vi "Litho objects manager.vi"() -> ()   [LabVIEW 2016]
uses:
  D:/Labview/Yang Hu/nanowriting_Akash/subVIs/Global Variables.vi
panel:
  in  "Cluster 2":T1
  in  "Cluster":T2
  in  "OK":bool
  in  "error in (no error)":errorcluster
  in  "Object index":string[](array[string])=["p6"]
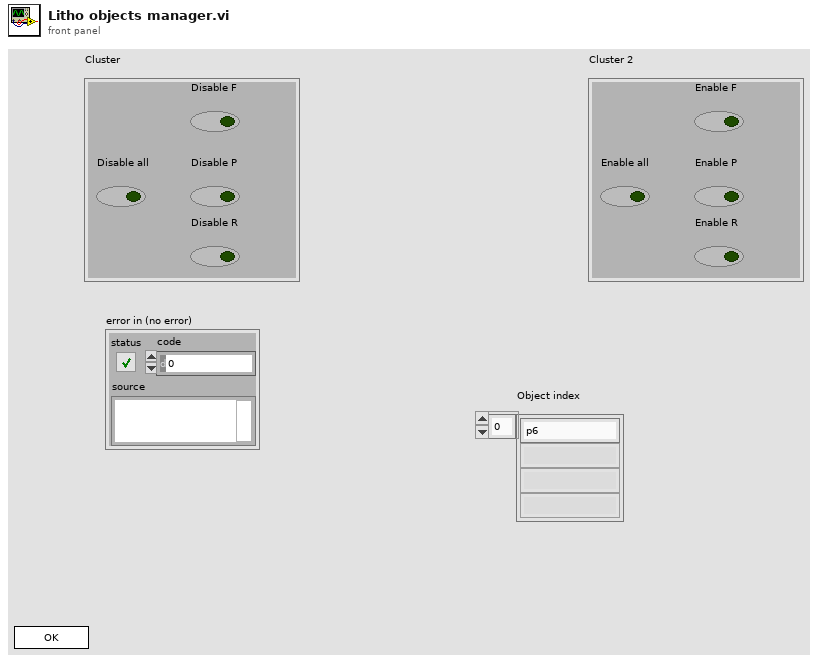
[diagram p1: front panel]
types:
  T1 = cluster{"Enable all":bool, "Enable F":bool, "Enable P":bool, "Enable R":bool}
  T2 = cluster{"Disable all":bool, "Disable F":bool, "Disable P":bool, "Disable R":bool}
  T3 = typedef "Funnel Properties - cluster.ctl" = cluster{"Enabled":bool, "Direction":u16, "Smooth Segments":dbl, "Bottom Segs.":dbl, "Speed (um/s)":T4, "Voltage (V)":T4, "Set Resistance":T7}
  T4 = typedef "Voltage - cluster.ctl" = cluster{"Schedule":T5, "Value":dbl, "Start Value":dbl, "End Value":dbl, "Min Value":dbl, "Max Value":dbl, "Duty Cycle (%)":dbl, "Signal Type":T6, "Cycle Number":dbl, "Phase (degrees)":dbl, "formula":string, "formula length (nm)":dbl, "formula resolution (nm)":dbl}
  T5 = typedef "Schedule - enum.ctl" = enum16{"Constant", "Ramp", "Fn. Generator", "Formula"}
  T6 = typedef "Signal Type - enum.ctl" = enum16{"Sine Wave", "Triangle Wave", "Square Wave", "Sawtooth Wave"}
  T7 = typedef "Resistor--enum.ctl" = enum16{"open", "discharge tip", "0 ohms", "100k ohm", "10M ohm", "1G ohm"}
  T8 = typedef "Path Properties - cluster.ctl" = cluster{"Enabled":bool, "Direction":u16, "Fill Orientation":u16, "Smooth Segments":dbl, "Fill Spacing":dbl, "Speed (um/s)":T4, "Voltage (V)":T4, "Set Resistance":T7}
  T9 = typedef "Rectangle Properties - cluster.ctl" = cluster{"Enabled":bool, "Direction":u16, "Fill Orientation":u16, "Fill Spacing":dbl, "Speed (um/s)":T4, "Voltage (V)":T4, "Set Resistance":T7}
  T10 = enum32{"Invalid", "Standard", "Closed", "Hidden", "Minimized", "Maximized"}
  T11 = enum32{"invalid app kind", "Development System", "Run Time System", "Student Edition", "Embedded LabVIEW", "Evaluation", "Custom"}
  T12 = cluster{"Core":cluster{"Current VI Reference":refnum<vi>, "Close Panel on Exit?":bool}, "Your Boolean data":bool, "Your string data":string}
  T13 = cluster{"Current VI Reference":refnum<vi>, "Close Panel on Exit?":bool}
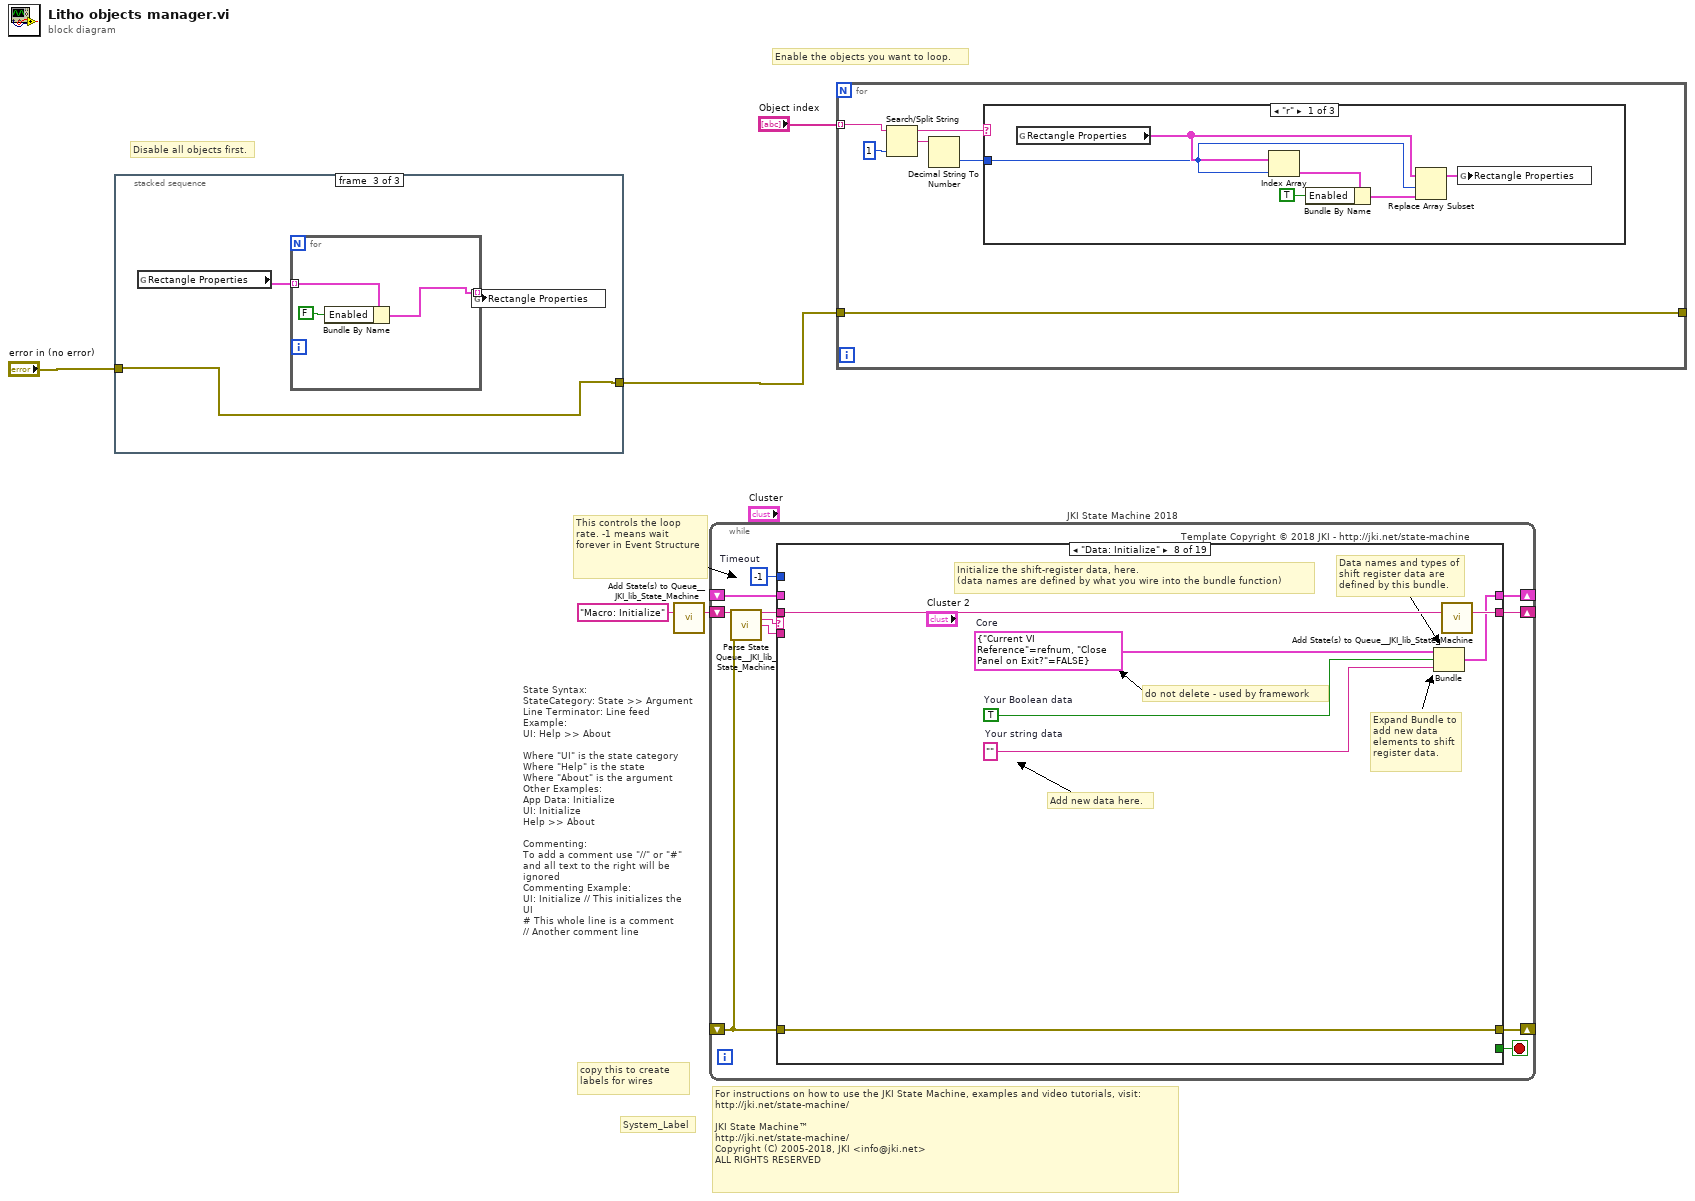
[diagram p0: block diagram]
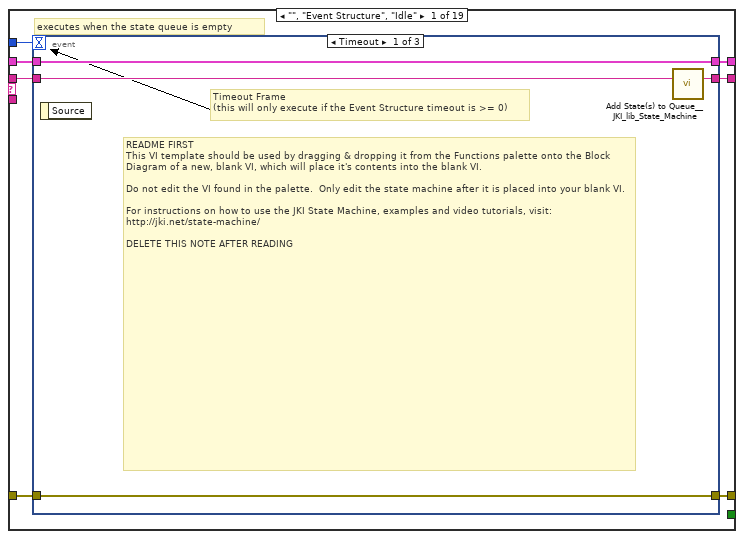
[diagram p2: hidden frame]
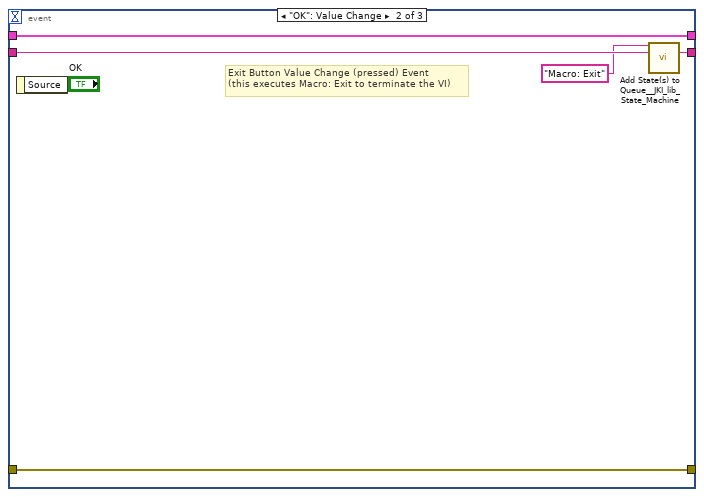
[diagram p3: hidden frame]
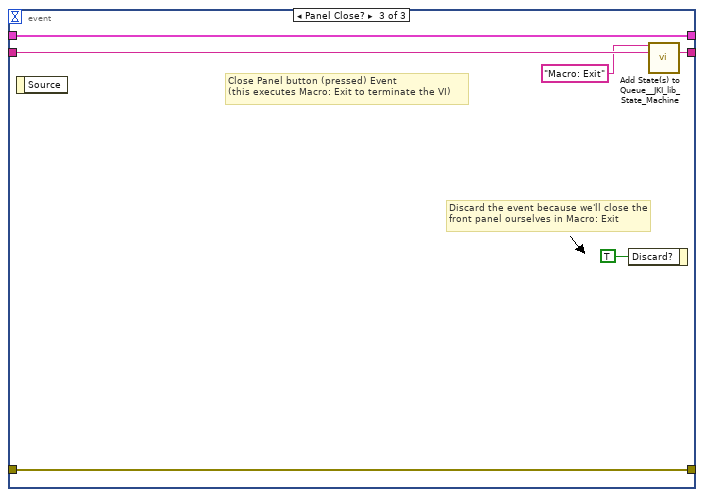
[diagram p4: hidden frame]
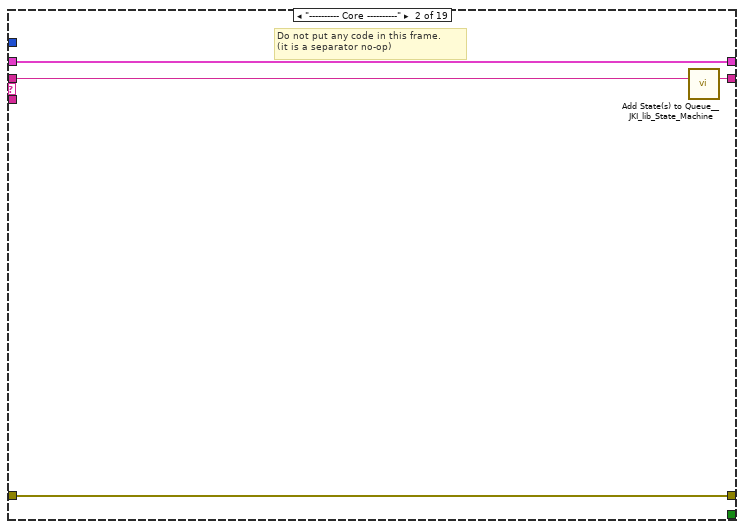
[diagram p5: hidden frame]
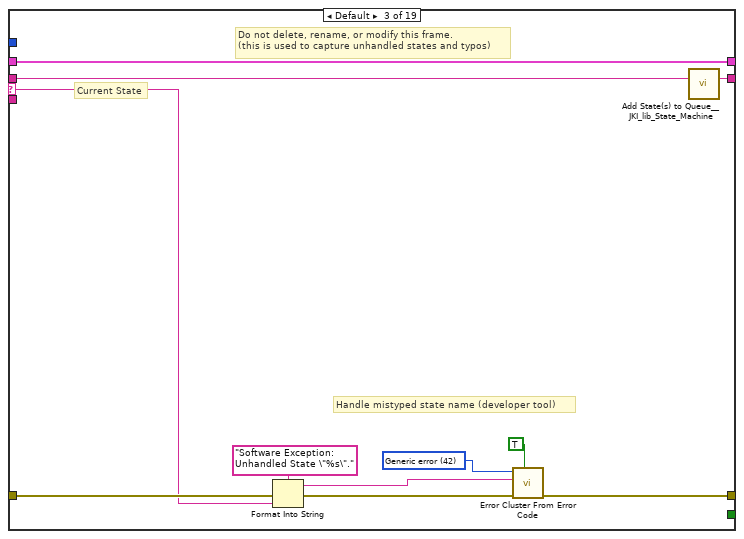
[diagram p6: hidden frame]
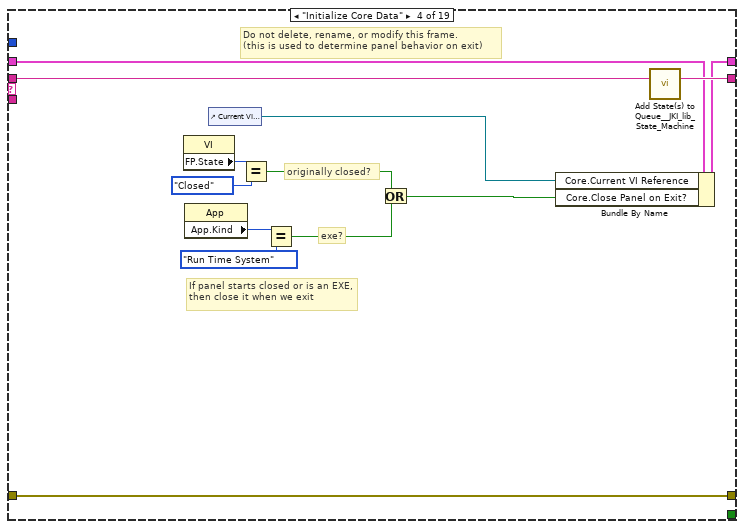
[diagram p7: hidden frame]
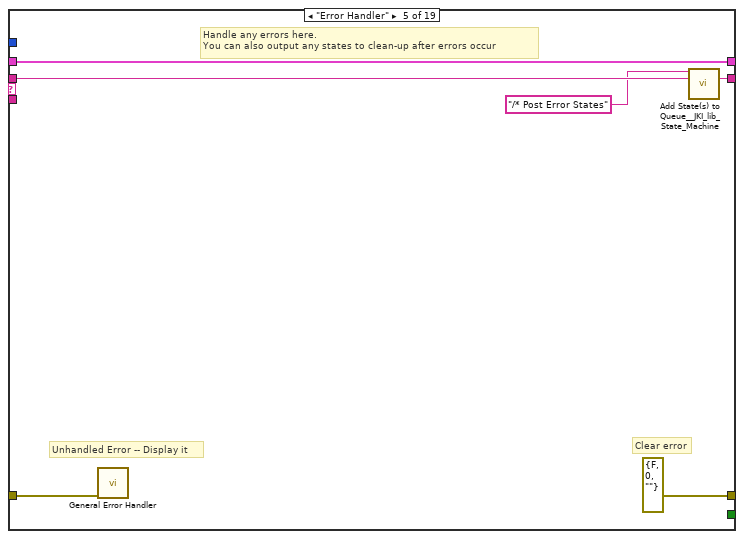
[diagram p8: hidden frame]
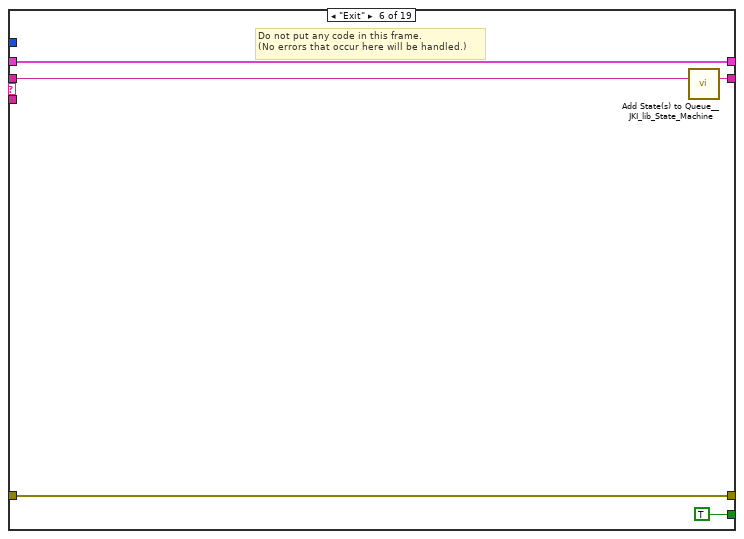
[diagram p9: hidden frame]
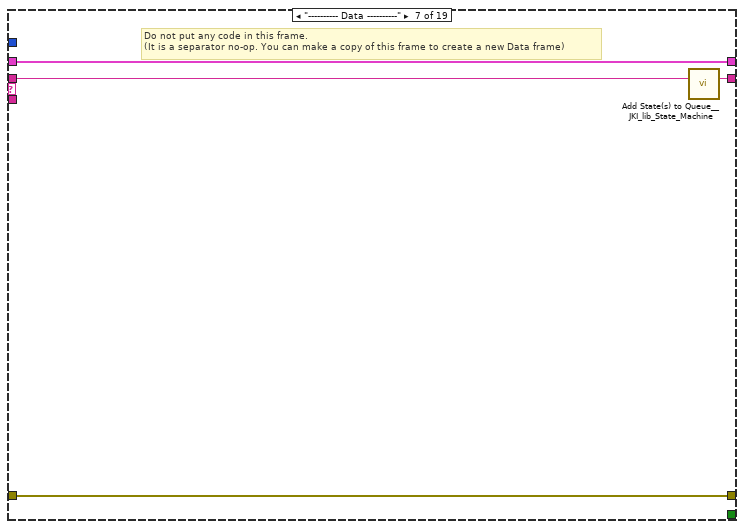
[diagram p10: hidden frame]
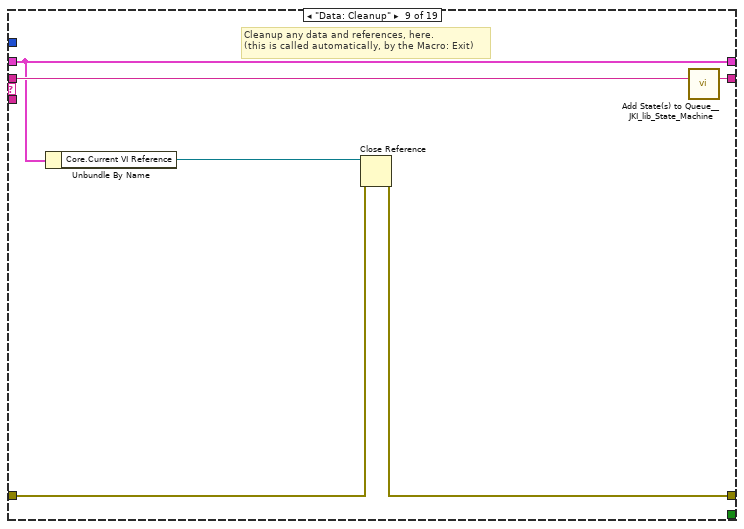
[diagram p11: hidden frame]
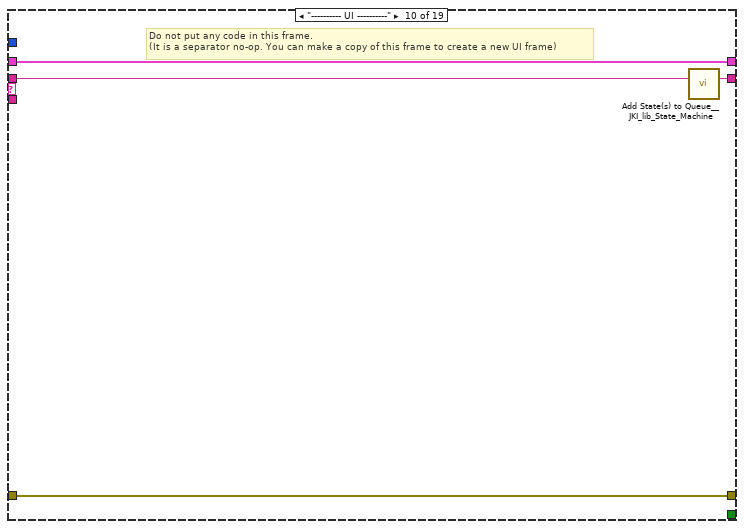
[diagram p12: hidden frame]
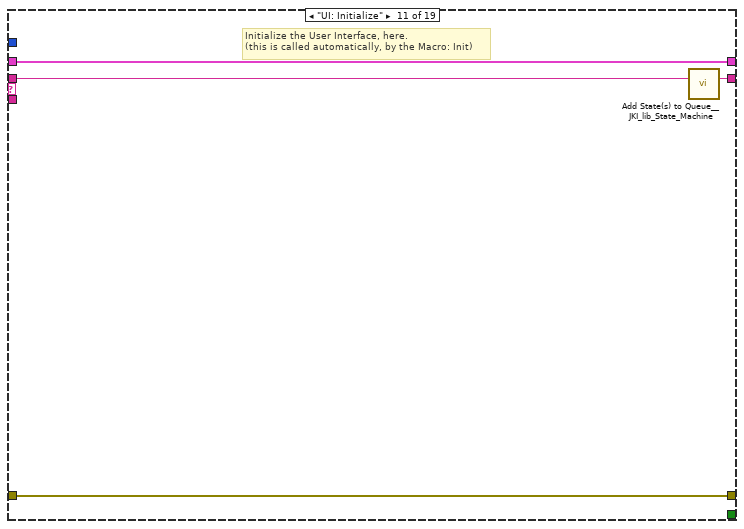
[diagram p13: hidden frame]
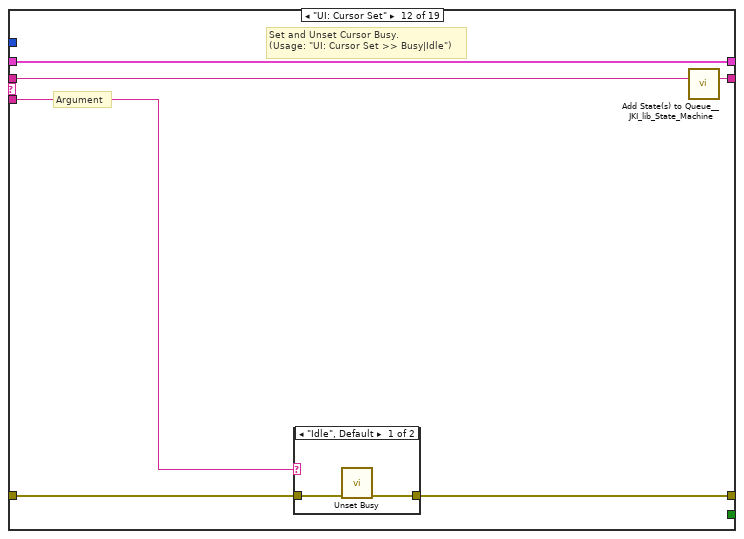
[diagram p14: hidden frame]
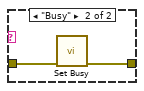
[diagram p15: hidden frame]
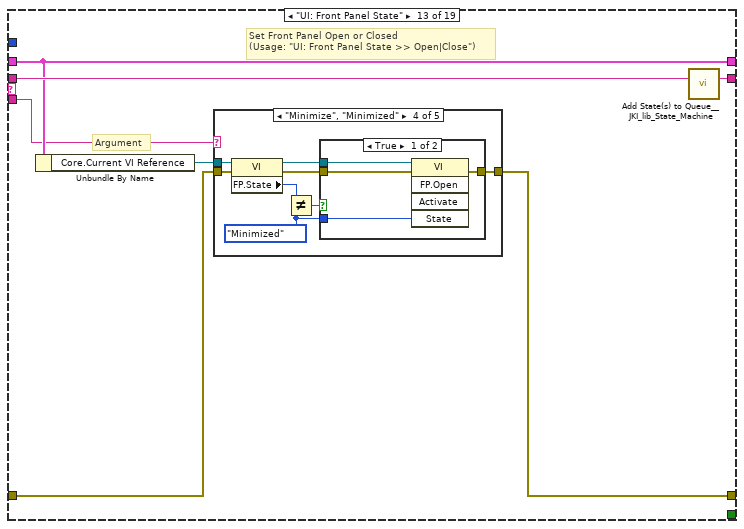
[diagram p16: hidden frame]
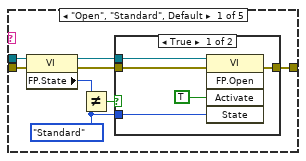
[diagram p17: hidden frame]
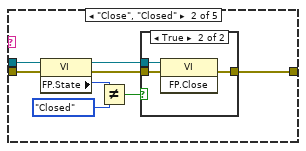
[diagram p19: hidden frame]
diagram:
  # "For instructions on how to use the JKI State Machine, examples and video tutorials, visit:\nhttp://jki.net/state-machine/\n\nJKI State Machine™\nhttp://jki.net/state-machine/\nCopyright (C) 2005-2018, JKI <info@jki.net>\nALL RIGHTS RESERVED"
  # "State Syntax:\nStateCategory: State >> Argument\nLine Terminator: Line feed\nExample:\nUI: Help >> About\n\nWhere \"UI\" is the state category\nWhere \"Help\" is the state\nWhere \"About\" is the argument\nOther Examples:\nApp Data: Initialize\nUI: Initialize\nHelp >> About\n\nCommenting:\nTo add a comment use \"//\" or \"#\" and all text to the right will be ignored\nCommenting Example:\nUI: Initialize // This initializes the UI\n# This whole line is a comment\n// Another comment line"
  # "copy this to create labels for wires"
  # "This controls the loop rate. -1 means wait forever in Event Structure"
  # "System_Label"
  # "Disable all objects first."
  # "Enable the objects you want to loop."
  n1 = stacked-sequence {
    tunnel: "error in (no error)" -> [_ _ w16]
    tunnel: [_ _ w16] -> w3
    frame #0 {
      n2 = global read "Global Variables.vi" "Funnel Properties"() -> (w6:T3[])
      n3 = for {
        tunnel: w6 -> [w9] mode=indexing
        tunnel: [w8] -> w7 mode=indexing
        n4 = Bundle By Name(cluster=w9, "Enabled"=FALSE) -> (w8:T3)
      }
      n5 = global write "Global Variables.vi" "Funnel Properties"(w7) -> ()
    }
    frame #1 {
      n6 = global read "Global Variables.vi" "Path Properties"() -> (w11:T8[])
      n7 = for {
        tunnel: w11 -> [w14] mode=indexing
        tunnel: [w13] -> w12 mode=indexing
        n8 = Bundle By Name(cluster=w14, "Enabled"=FALSE) -> (w13:T8)
      }
      n9 = global write "Global Variables.vi" "Path Properties"(w12) -> ()
    }
    frame #2 {
      n10 = global read "Global Variables.vi" "Rectangle Properties"() -> (w17:T9[])
      n11 = for {
        tunnel: w17 -> [w20] mode=indexing
        tunnel: [w19] -> w18 mode=indexing
        n12 = Bundle By Name(cluster=w20, "Enabled"=FALSE) -> (w19:T9)
      }
      n13 = global write "Global Variables.vi" "Rectangle Properties"(w18) -> ()
    }
  }
  n14 = call <vilib>:"Add State(s) to Queue__JKI_lib_State_Machine.vi"("State(s) in (\"\")"="Macro: Initialize") -> ("States Out"=w2:string)  [unwired: 14 in]
  n15 = while "JKI State Machine 2018" {
    shift-right: [w25] -> _
    shift-left: _ -> [w24]
    shift-right: [w28] -> _
    shift-left: _ -> [w22]
    shift-right: [w27] -> _
    shift-left: w2 -> [w29]
    stop <- w26 stop-if-true
    w23 = -1  # Timeout
    # "Template Copyright © 2018 JKI - http://jki.net/state-machine"
    n16 = call <vilib>:"Parse State Queue__JKI_lib_State_Machine.vi"("State Queue"=w29, "Error In (no error)"=w22) -> ("Remaining States"=w31:string, "Current State"=w32:string, "Arguments"=w30:string)  [unwired: 11 in]
    n17 = case shown="\"Data: Initialize\"" w32 {
      selector: w32 -> [_ _ w59 _ _ _ _ _ _ _ _ _ _ _ _ _ _ _ _]
      tunnel: w31 -> [w39 w58 w63 w82 w88 w93 w97 w104 w110 w114 w118 w124 w135 w204 w209 w219 w223 w227 w231]
      tunnel: w30 -> [_ _ _ _ _ _ _ _ _ _ _ w119 w129 _ _ _ _ _ _]
      tunnel: w24 -> [w37 w55 w61 w75 w85 w91 w94 _ w105 w111 w116 w122 w131 w201 w206 w216 w220 w224 w228]
      tunnel: [w36 w56 w65 w79 errorcluster {"status"=FALSE, "code"=0, "source"=""} ("error out") w90 w95 w101 w106 w112 w115 w120 w132 w202 w207 w217 w221 w225 w229] -> w28
      tunnel: w22 -> [w35 w56 w64 w79 w84 w90 w95 w101 w107 w112 w115 w121 w133 w202 w207 w217 w221 w225 w229]
      tunnel: [w38 w57 w62 w81 w87 w92 w96 w103 w109 w113 w117 w123 w134 w203 w208 w218 w222 w226 w230] -> w27
      tunnel: [_ _ _ _ _ TRUE _ _ _ _ _ _ _ _ _ _ _ _ _] -> w26
      tunnel: [w34 w55 w61 w80 w85 w91 w94 w102 w105 w111 w116 w122 w131 w201 w206 w216 w220 w224 w228] -> w25
      tunnel: w23 -> [w33 _ _ _ _ _ _ _ _ _ _ _ _ _ _ _ _ _ _]
      frame "", "Event Structure", "Idle" {
        # "executes when the state queue is empty"
        n18 = event shown="[0] Timeout" {
          selector: _ -> [_ _ _]
          dyn-events: _ -> [_ _ _]
          timeout: w33 -> [_ _ _]
          tunnel: w39 -> [w43 w48 w54]
          tunnel: [w42 w47 w53] -> w38
          tunnel: w37 -> [w40 w45 w51]
          tunnel: [w41 w46 w52] -> w36
          tunnel: w35 -> [w41 w46 w52]
          tunnel: [w40 w45 w51] -> w34
          event Timeout {
            # "README FIRST\nThis VI template should be used by dragging & dropping it from the Functions palette onto the Block Diagram of a new, blank VI, which will place it's contents into the blank VI.\n\nDo not edit the VI found in the palette.  Only edit the state machine after it is placed into your blank VI.\n\nFor instructions on how to use the JKI State Machine, examples and video tutorials, visit:\nhttp://jki.net/state-machine/\n\nDELETE THIS NOTE AFTER READING"
            # "Timeout Frame\n(this will only execute if the Event Structure timeout is >= 0)"
            n19 = event-data() -> ()  [unwired: 1 in, 1 out]
            n20 = call <vilib>:"Add State(s) to Queue__JKI_lib_State_Machine.vi"("State(s) in (\"\")"=w43) -> ("States Out"=w42:string)  [unwired: 14 in]
          }
          event "OK": Value Change {
            # "Exit Button Value Change (pressed) Event\n(this executes Macro: Exit to terminate the VI)"
            n21 = event-data() -> ()  [unwired: 1 in, 1 out]
            n22 = call <vilib>:"Add State(s) to Queue__JKI_lib_State_Machine.vi"("State(s) in Front (\"\")"="Macro: Exit", "State(s) in (\"\")"=w48) -> ("States Out"=w47:string)  [unwired: 13 in]
          }
          event Panel Close? {
            # "Discard the event because we'll close the front panel ourselves in Macro: Exit"
            # "Close Panel button (pressed) Event\n(this executes Macro: Exit to terminate the VI)"
            n23 = event-data() -> ()  [unwired: 1 in, 1 out]
            n24 = event-data("Discard?"=TRUE) -> ()  [unwired: 1 in, 1 out]
            n25 = call <vilib>:"Add State(s) to Queue__JKI_lib_State_Machine.vi"("State(s) in Front (\"\")"="Macro: Exit", "State(s) in (\"\")"=w54) -> ("States Out"=w53:string)  [unwired: 13 in]
          }
        }
      }
      frame "---------- Core ----------" {
        # "Do not put any code in this frame.\n(it is a separator no-op)"
        n26 = call <vilib>:"Add State(s) to Queue__JKI_lib_State_Machine.vi"("State(s) in (\"\")"=w58) -> ("States Out"=w57:string)  [unwired: 14 in]
      }
      frame Default {
        w68 = 42 items=["No error", "Argument error", "Memory is full", "Out of zone", "End of file", "File already open", "Generic file I/O error", "File not found", "File permission error", "Disk is full", "Duplicate path", "Too many files open", "System feature not enabled", "Resource file not found", "Cannot add resource", "Resource not found", "Image not found", "Image memory error", "Pen does not exist", "Config type invalid", "Config token not found", "Config parse error", "Config memory error", "Bad external code format", "Bad external code offset", "External code not present", "Null window", "Destroy window error", "Null menu", "Print aborted", "Bad print record", "Print driver error", "Windows error during printing", "Memory error during printing", "Print dialog error", "Generic print error", "Invalid device refnum", "Device not found", "Device parameter error", "Device unit error", "Cannot open device", "Device call aborted", "Generic error", "Cancelled by user", "Object ID too low", "Object ID too high", "Object not in heap", "Unknown heap", "Unknown object (invalid DefProc)", "Unknown object (DefProc not in table)", "Message out of range", "Invalid (null) method", "Unknown message", "Manager call not supported", "Bad address", "Network operation in progress", "Network operation timed out", "Connection is busy", "Network attribute not supported", "Network error", "Address in use", "System out of memory", "Connection aborted", "Connection refused", "Not connected", "Already connected", "Connection closed", "Initialization error (interapplication manager)", "Bad occurrence", "Wait on unbound occurrence handler", "Occurrence queue overflow", "Datalog type conflict", "Unused", "Unrecognized type (interapplication manager)", "Memory corrupt", "Failed to make temporary DLL", "Old CIN version", "Drag socket not found", "Failed to load drop-object", "Failed to register OLE object", "Failed to release OLE object", "Format specifier type mismatch", "Unknown format specifier", "Too few format specifiers", "Too many format specifiers", "Scan failed", "Newer CIN version", "Error converting to variant", "Runtime menu error", "Password tampered", "Variant attribute not found", "Incompatible variant data type", "Event data is not available", "Event Store is not present", "Occurrence is not found", "Event Queue is not created", "Event info is not available", "Refnum passed is NULL", "Error retrieving Class GUID", "Error retrieving CoClass GUID", "Error retrieving TypeLib GUID.", "Bad built application magic bytes.", "Specific driver is different from the specific driver associated with the Logical Name.", "There is no session opened to the class driver.", "Max Error", "MAX - Error with config objects", "MAX - Error loading configuration", "MAX - Group not supported"]
        # "Current State"
        # "Do not delete, rename, or modify this frame.\n(this is used to capture unhandled states and typos)"
        # "Handle mistyped state name (developer tool)"
        n27 = Format Into String(format string="Software Exception: Unhandled State \"%s\"." ("message"), error in=w64, w59) -> (resulting string=w67:string, error out=w66:errorcluster)  [unwired: 1 in]
        n28 = call <vilib>:"Error Cluster From Error Code.vi"("show call chain? (False)"=TRUE, "error in (no error)"=w66, "error message (\"\")"=w67, "error code (0)"=w68) -> ("error out"=w65:errorcluster)  [unwired: 5 in]
        n29 = call <vilib>:"Add State(s) to Queue__JKI_lib_State_Machine.vi"("State(s) in (\"\")"=w63) -> ("States Out"=w62:string)  [unwired: 14 in]
      }
      frame "Initialize Core Data" {
        # "Do not delete, rename, or modify this frame.\n(this is used to determine panel behavior on exit)"
        # "originally closed?"
        # "exe?"
        # "If panel starts closed or is an EXE, then close it when we exit"
        n30 = property class="VI"() -> ("FP.State"=w72:T10)  [unwired: 2 in, 2 out]
        n31 = property class="App"() -> ("App.Kind"=w78:T11)  [unwired: 2 in, 2 out]
        n32 = control-ref of="Current VI Reference"() -> (w73:refnum<vi>)
        n33 = Equal?(x=w72, y=T10."Closed" ("Front Panel Window:State")) -> (x = y?=w70:bool)
        n34 = Equal?(x=w78, y=T11."Run Time System" ("Application:Kind")) -> (x = y?=w76:bool)
        n35 = Or(x=w70, y=w76) -> (x .or. y?=w74:bool)
        n36 = Bundle By Name(cluster=w75, "Core.Current VI Reference"=w73, "Core.Close Panel on Exit?"=w74) -> (w80:T12)
        n37 = call <vilib>:"Add State(s) to Queue__JKI_lib_State_Machine.vi"("State(s) in (\"\")"=w82) -> ("States Out"=w81:string)  [unwired: 14 in]
      }
      frame "Error Handler" {
        # "Unhandled Error -- Display it"
        # "Handle any errors here.\nYou can also output any states to clean-up after errors occur"
        # "Clear error"
        n38 = call <vilib>:"General Error Handler.vi"("error in (no error)"=w84) -> ()  [unwired: 10 in, 5 out]
        n39 = call <vilib>:"Add State(s) to Queue__JKI_lib_State_Machine.vi"("State(s) in Front (\"\")"="/* Post Error States", "State(s) in (\"\")"=w88) -> ("States Out"=w87:string)  [unwired: 13 in]
      }
      frame "Exit" {
        # "Do not put any code in this frame.\n(No errors that occur here will be handled.)"
        n40 = call <vilib>:"Add State(s) to Queue__JKI_lib_State_Machine.vi"("State(s) in (\"\")"=w93) -> ("States Out"=w92:string)  [unwired: 14 in]
      }
      frame "---------- Data ----------" {
        # "Do not put any code in this frame.\n(It is a separator no-op. You can make a copy of this frame to create a new Data frame)"
        n41 = call <vilib>:"Add State(s) to Queue__JKI_lib_State_Machine.vi"("State(s) in (\"\")"=w97) -> ("States Out"=w96:string)  [unwired: 14 in]
      }
      frame "Data: Initialize" {
        w98 = T13 {"Current VI Reference"=refnum, "Close Panel on Exit?"=FALSE}  # Core
        w100 = TRUE  # Your Boolean data
        w99 = ""  # Your string data
        # "do not delete - used by framework"
        # "Expand Bundle to add new data elements to shift register data."
        # "Add new data here."
        # "Data names and types of shift register data are defined by this bundle."
        # "Initialize the shift-register data, here.\n(data names are defined by what you wire into the bundle function)"
        n42 = Bundle("Core"=w98, "Your Boolean data"=w100, "Your string data"=w99) -> (w102:T12)  [unwired: 1 in]
        n43 = call <vilib>:"Add State(s) to Queue__JKI_lib_State_Machine.vi"("State(s) in (\"\")"=w104) -> ("States Out"=w103:string)  [unwired: 14 in]
      }
      frame "Data: Cleanup" {
        # "Cleanup any data and references, here.\n(this is called automatically, by the Macro: Exit)"
        n44 = Unbundle By Name(w105) -> ("Core.Current VI Reference"=w108:refnum<vi>)
        n45 = Close Reference(reference=w108, error in (no error)=w107) -> (error out=w106:errorcluster)
        n46 = call <vilib>:"Add State(s) to Queue__JKI_lib_State_Machine.vi"("State(s) in (\"\")"=w110) -> ("States Out"=w109:string)  [unwired: 14 in]
      }
      frame "---------- UI ----------" {
        # "Do not put any code in this frame.\n(It is a separator no-op. You can make a copy of this frame to create a new UI frame)"
        n47 = call <vilib>:"Add State(s) to Queue__JKI_lib_State_Machine.vi"("State(s) in (\"\")"=w114) -> ("States Out"=w113:string)  [unwired: 14 in]
      }
      frame "UI: Initialize" {
        # "Initialize the User Interface, here.\n(this is called automatically, by the Macro: Init)"
        n48 = call <vilib>:"Add State(s) to Queue__JKI_lib_State_Machine.vi"("State(s) in (\"\")"=w118) -> ("States Out"=w117:string)  [unwired: 14 in]
      }
      frame "UI: Cursor Set" {
        # "Argument"
        # "Set and Unset Cursor Busy.\n(Usage: \"UI: Cursor Set >> Busy|Idle\")"
        n49 = case shown="\"Idle\", Default" w119 {
          tunnel: w121 -> [w126 w128]
          tunnel: [w125 w127] -> w120
          frame "Idle", Default {
            n50 = call <vilib>:"Unset Busy.vi"("error in (no error)"=w126) -> ("error out"=w125:errorcluster)  [unwired: 10 in]
          }
          frame "Busy" {
            n51 = call <vilib>:"Set Busy.vi"("error in (no error)"=w128) -> ("error out"=w127:errorcluster)  [unwired: 9 in, 1 out]
          }
        }
        n52 = call <vilib>:"Add State(s) to Queue__JKI_lib_State_Machine.vi"("State(s) in (\"\")"=w124) -> ("States Out"=w123:string)  [unwired: 14 in]
      }
      frame "UI: Front Panel State" {
        # "Argument"
        # "Set Front Panel Open or Closed\n(Usage: \"UI: Front Panel State >> Open|Close\")"
        n53 = Unbundle By Name(w131) -> ("Core.Current VI Reference"=w130:refnum<vi>)
        n54 = case shown="\"Minimize\", \"Minimized\"" w129 {
          tunnel: w133 -> [w141 w156 w167 w180 w193]
          tunnel: [w143 w157 w169 w182 w195] -> w132
          tunnel: w130 -> [w142 w154 w168 w181 w194]
          frame "Open", "Standard", Default {
            w136 = T10."Standard" ("State")
            n55 = property class="VI"(reference=w142, error in=w141) -> (reference out=w139:refnum<vi>, error out=w140:errorcluster, "FP.State"=w138:T10)
            n56 = Not Equal?(x=w138, y=w136) -> (x != y?=w137:bool)
            n57 = case shown="True" w137 {
              tunnel: [w147 w149] -> w143
              tunnel: w140 -> [w146 w149]
              tunnel: w139 -> [w145 _]
              tunnel: w136 -> [w144 _]
              frame True {
                n58 = invoke class="VI" method="FP.Open"(reference=w145, error in=w146, "Activate"=TRUE, "State"=w144) -> (error out=w147:errorcluster)  [unwired: 1 in, 4 out]
              }
              frame False {
              }
            }
          }
          frame "Close", "Closed" {
            n59 = property class="VI"(reference=w154, error in=w156) -> (reference out=w153:refnum<vi>, error out=w155:errorcluster, "FP.State"=w151:T10)
            n60 = Not Equal?(x=w151, y=T10."Closed" ("Front Panel Window:State")) -> (x != y?=w150:bool)
            n61 = case shown="True" w150 {
              tunnel: [w158 w161] -> w157
              tunnel: w155 -> [w158 w160]
              tunnel: w153 -> [_ w159]
              frame False {
              }
              frame True {
                n62 = invoke class="VI" method="FP.Close"(reference=w159, error in=w160) -> (error out=w161:errorcluster)  [unwired: 1 in, 2 out]
              }
            }
          }
          frame "Hidden", "Hide" {
            w162 = T10."Hidden" ("State")
            n63 = property class="VI"(reference=w168, error in=w167) -> (reference out=w165:refnum<vi>, error out=w166:errorcluster, "FP.State"=w164:T10)
            n64 = Not Equal?(x=w164, y=w162) -> (x != y?=w163:bool)
            n65 = case shown="True" w163 {
              tunnel: [w173 w174] -> w169
              tunnel: w166 -> [w172 w174]
              tunnel: w165 -> [w171 _]
              tunnel: w162 -> [w170 _]
              frame True {
                n66 = invoke class="VI" method="FP.Open"(reference=w171, error in=w172, "State"=w170) -> (error out=w173:errorcluster)  [unwired: 2 in, 4 out]
              }
              frame False {
              }
            }
          }
          frame "Minimize", "Minimized" {
            w175 = T10."Minimized" ("State")
            n67 = property class="VI"(reference=w181, error in=w180) -> (reference out=w178:refnum<vi>, error out=w179:errorcluster, "FP.State"=w177:T10)
            n68 = Not Equal?(x=w177, y=w175) -> (x != y?=w176:bool)
            n69 = case shown="True" w176 {
              tunnel: [w186 w187] -> w182
              tunnel: w179 -> [w185 w187]
              tunnel: w178 -> [w184 _]
              tunnel: w175 -> [w183 _]
              frame True {
                n70 = invoke class="VI" method="FP.Open"(reference=w184, error in=w185, "State"=w183) -> (error out=w186:errorcluster)  [unwired: 2 in, 4 out]
              }
              frame False {
              }
            }
          }
          frame "Maximize", "Maximized" {
            w188 = T10."Maximized" ("State")
            n71 = property class="VI"(reference=w194, error in=w193) -> (reference out=w191:refnum<vi>, error out=w192:errorcluster, "FP.State"=w190:T10)
            n72 = Not Equal?(x=w190, y=w188) -> (x != y?=w189:bool)
            n73 = case shown="True" w189 {
              tunnel: [w199 w200] -> w195
              tunnel: w192 -> [w198 w200]
              tunnel: w191 -> [w197 _]
              tunnel: w188 -> [w196 _]
              frame True {
                n74 = invoke class="VI" method="FP.Open"(reference=w197, error in=w198, "State"=w196) -> (error out=w199:errorcluster)  [unwired: 2 in, 4 out]
              }
              frame False {
              }
            }
          }
        }
        n75 = call <vilib>:"Add State(s) to Queue__JKI_lib_State_Machine.vi"("State(s) in (\"\")"=w135) -> ("States Out"=w134:string)  [unwired: 14 in]
      }
      frame "---------- Macro ----------" {
        # "Do not put any code in this frame.\n(It is a separator no-op. You can make a copy of this frame to create a new Macro frame)"
        n76 = call <vilib>:"Add State(s) to Queue__JKI_lib_State_Machine.vi"("State(s) in (\"\")"=w204) -> ("States Out"=w203:string)  [unwired: 14 in]
      }
      frame "Macro: Initialize" {
        w205 = "Data: Initialize\nInitialize Core Data\nUI: Initialize\nUI: Front Panel State >> Open"  # Data: Initialize Initialize Core Data UI: Initialize UI: Front Panel State >> Open
        # "Initialization Macro\n(This is called once, when the VI starts)"
        n77 = call <vilib>:"Add State(s) to Queue__JKI_lib_State_Machine.vi"("State(s) in Front (\"\")"=w205, "State(s) in (\"\")"=w209) -> ("States Out"=w208:string)  [unwired: 13 in]
      }
      frame "Macro: Exit" {
        # "Exit Macro\n(This is called once, when the VI exits)"
        n78 = Unbundle By Name(w216) -> ("Core.Close Panel on Exit?"=w215:bool)
        n79 = Select(t="UI: Front Panel State >> Close", s=w215, f="") -> (s? t:f=w212:string)
        n80 = call <vilib>:"Add State(s) to Queue__JKI_lib_State_Machine.vi"("State(s) in (\"\")"=w212, "State(s) at Back (\"\")"="Data: Cleanup\nExit") -> ("States Out"=w210:string)  [unwired: 13 in]
        n81 = call <vilib>:"Add State(s) to Queue__JKI_lib_State_Machine.vi"("State(s) in Front (\"\")"=w210, "State(s) in (\"\")"=w219) -> ("States Out"=w218:string)  [unwired: 13 in]
      }
      frame "---------- New Category ----------" {
        # "Template Separator\n(You can make a copy of, or modify, this frame)"
        n82 = call <vilib>:"Add State(s) to Queue__JKI_lib_State_Machine.vi"("State(s) in (\"\")"=w223) -> ("States Out"=w222:string)  [unwired: 14 in]
      }
      frame "New Category: 1" {
        # "Your code here.\n(You can make a copy of, or modify, this frame)"
        n83 = call <vilib>:"Add State(s) to Queue__JKI_lib_State_Machine.vi"("State(s) in (\"\")"=w227) -> ("States Out"=w226:string)  [unwired: 14 in]
      }
      frame "New Category: 2" {
        # "Your code here.\n(You can make a copy of, or modify, this frame)"
        n84 = call <vilib>:"Add State(s) to Queue__JKI_lib_State_Machine.vi"("State(s) in (\"\")"=w231) -> ("States Out"=w230:string)  [unwired: 14 in]
      }
    }
  }
  n85 = for {
    tunnel: "Object index" -> [w233] mode=indexing
    tunnel: [w232] -> _
    tunnel: w3 -> [w232]
    n86 = Search/Split String(string=w233, offset (0)=1) -> (substring before match=w235:string, match + rest of string=w236:string)  [unwired: 1 in, 1 out]
    n87 = Decimal String To Number(string=w236) -> (number=w234:i32)  [unwired: 2 in, 1 out]
    n88 = case shown="\"r\"" w235 {
      tunnel: w234 -> [w238 w244 w250]
      frame "r" {
        n89 = global read "Global Variables.vi" "Rectangle Properties"() -> (w242:T9[])
        n90 = Index Array(array=w242, index=w238) -> (element=w239:T9)
        n91 = Bundle By Name(cluster=w239, "Enabled"=TRUE) -> (w240:T9)
        n92 = Replace Array Subset(array=w242, new element=w240, index=w238) -> (w243:T9[])
        n93 = global write "Global Variables.vi" "Rectangle Properties"(w243) -> ()
      }
      frame "p", Default {
        n94 = global read "Global Variables.vi" "Path Properties"() -> (w248:T8[])
        n95 = Index Array(array=w248, index=w244) -> (element=w245:T8)
        n96 = Bundle By Name(cluster=w245, "Enabled"=TRUE) -> (w246:T8)
        n97 = Replace Array Subset(array=w248, new element=w246, index=w244) -> (w249:T8[])
        n98 = global write "Global Variables.vi" "Path Properties"(w249) -> ()
      }
      frame "f" {
        n99 = global read "Global Variables.vi" "Funnel Properties"() -> (w254:T3[])
        n100 = Index Array(array=w254, index=w250) -> (element=w251:T3)
        n101 = Bundle By Name(cluster=w251, "Enabled"=TRUE) -> (w252:T3)
        n102 = Replace Array Subset(array=w254, new element=w252, index=w250) -> (w255:T3[])
        n103 = global write "Global Variables.vi" "Funnel Properties"(w255) -> ()
      }
    }
  }
